vi "final_lucas_valeria.vi"() -> ()   [LabVIEW 2017]
uses:
  <vilib>/ErrorRing/Error Ring.xnode
  final.ctl
  <vilib>/Utility/file.llb/Read Delimited Spreadsheet (string).vi
panel:
  out "Decodificar":string
  out "substring":string
  out "cabecera":bool
  out "x = y?":bool
  out "led3":bool
  out "led2":bool
  out "led1":bool
  in  "Umbral min3":dbl
  in  "Umbral max3":dbl
  in  "Umbral min2":dbl
  in  "Umbral max2":dbl
  in  "Umbral min1":dbl
  in  "Umbral max1":dbl
  out "pt100":dbl(knob) scale=0.0..100.0
  out "ntc":dbl(knob) scale=0.0..100.0
  out "lm35":dbl(knob) scale=0.0..150.0
  out "Waveform Chart":cluster{"lm35":dbl, "ntc":dbl}(graph)
  out "NTC":dbl=25.0 format="%0.2f"
  out "lM35":dbl
  out "Dato3":dbl
  out "Dato2":dbl
  out "verifica_cheacksum":string
  out "Dato_Act":string
  out "size":i32
  out "CHECKSUM":string
  out "Desconexión":bool
  out "Hora de desconexión":string
  out "Stop":bool
  in  "BaudRate":i32(ring) items=["9600"=9600, "11520"=11520]
  out "error out":errorcluster
  out "On":bool
  out "Recibiendo datos":bool
  out "Datos Sensores":string
  in  "Close":bool
  in  "Open":bool
  in  "Port":string(combo)
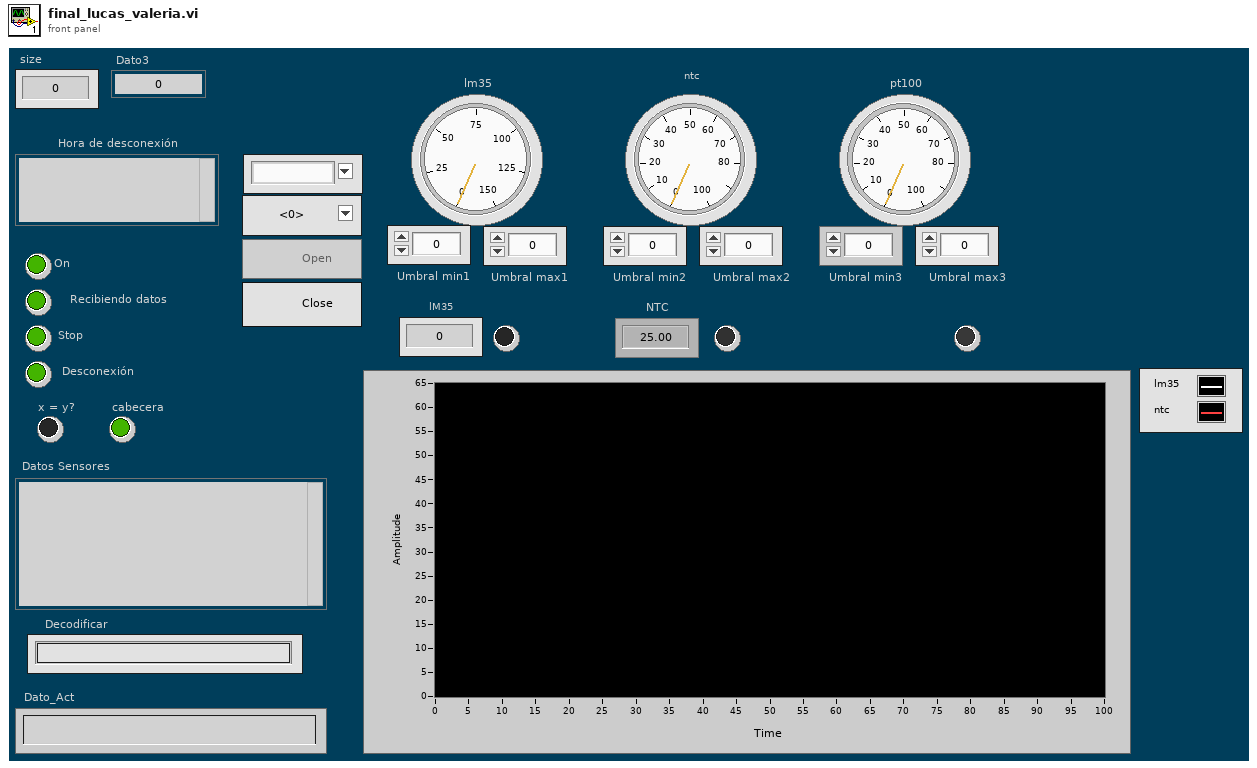
[diagram p1: front panel]
types:
  T1 = typedef "final.ctl" = enum16{"verificar", "verificar2", "sacar_datos", "alarma1", "alarma2", "alarma3"}
  T2 = enum8{"Enabled", "Disabled", "Disabled and Grayed Out"}
  T3 = enum16{"open", "replace", "create", "open or create", "replace or create", "replace or create with confirmation"}
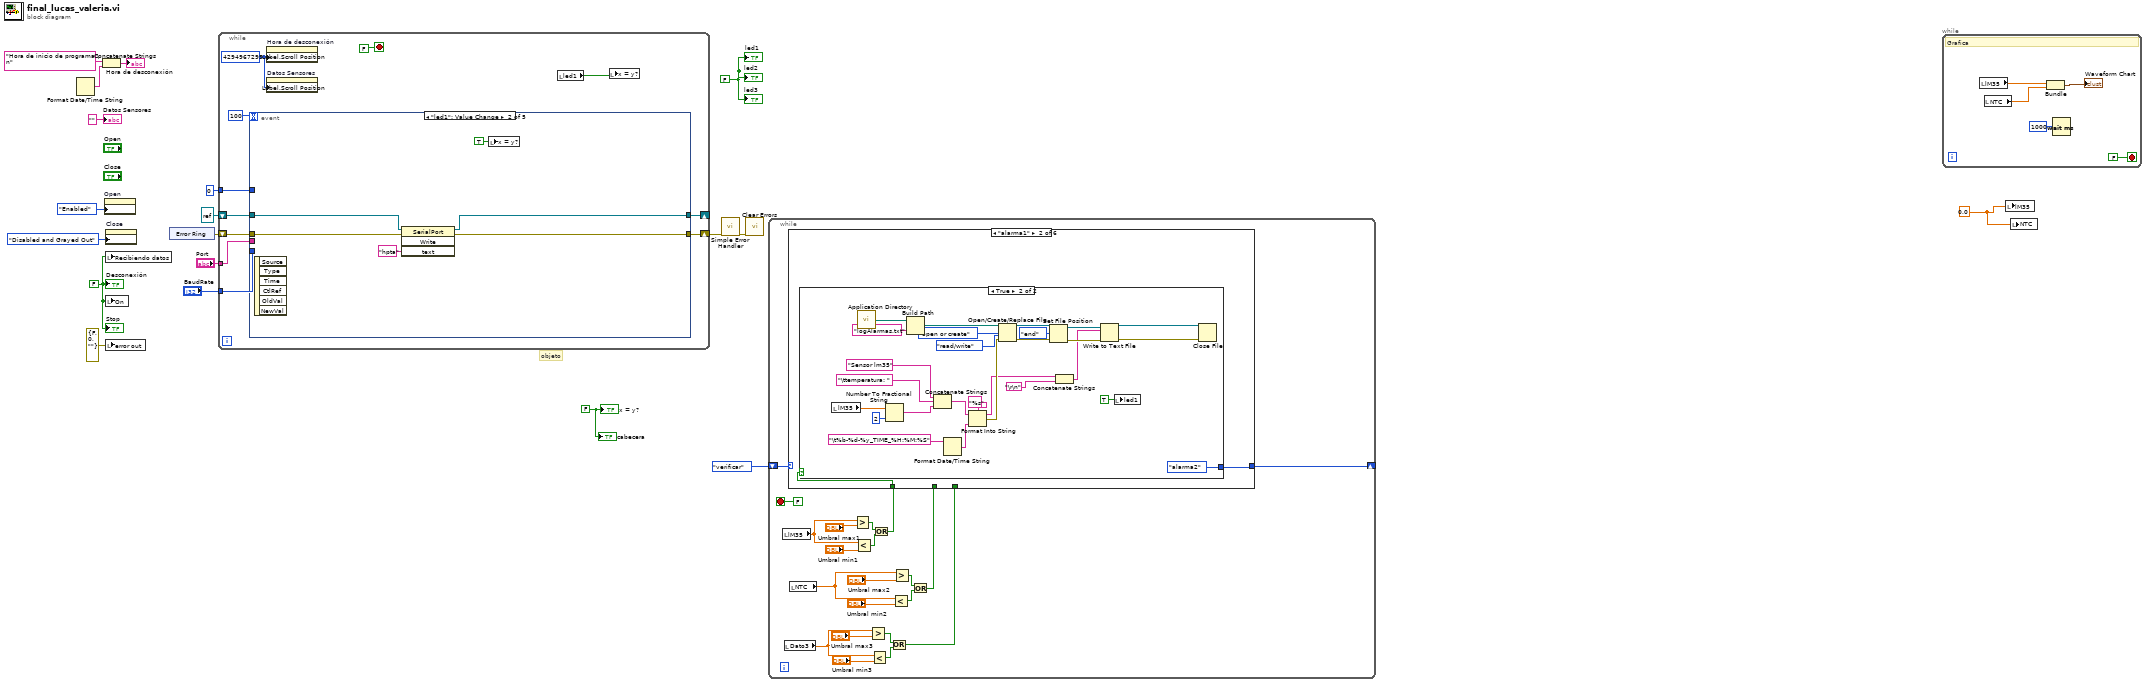
[diagram p0: block diagram]
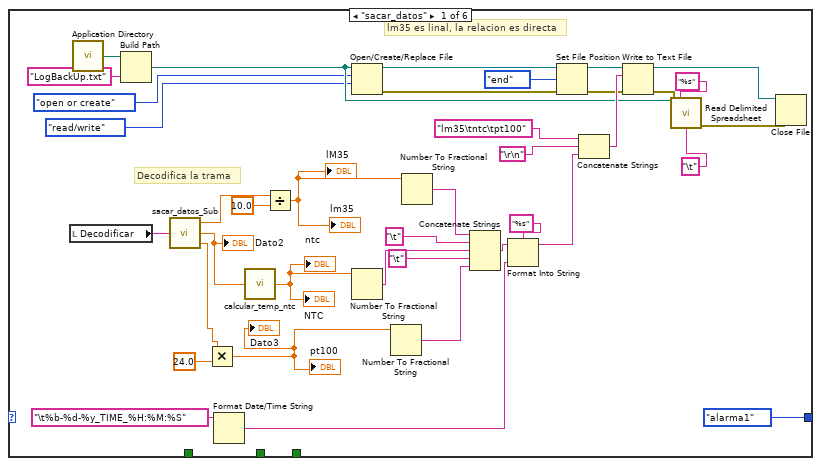
[diagram p2: hidden frame]
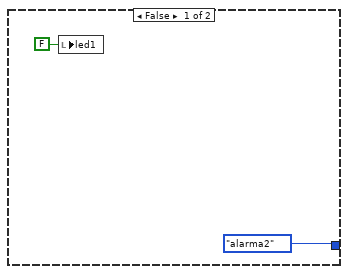
[diagram p3: hidden frame]
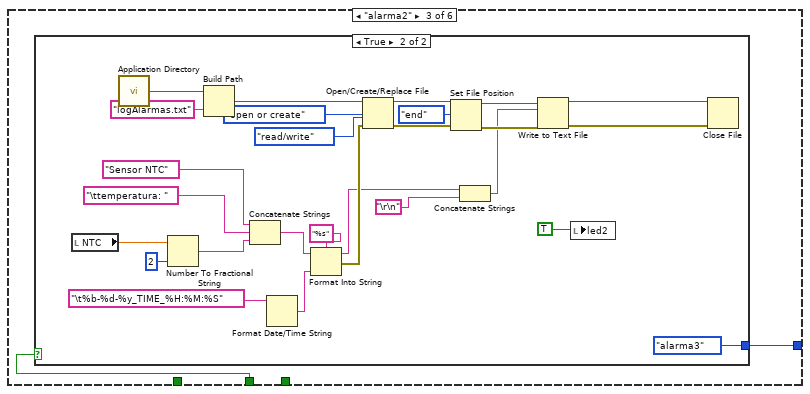
[diagram p4: hidden frame]
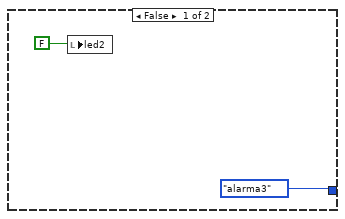
[diagram p5: hidden frame]
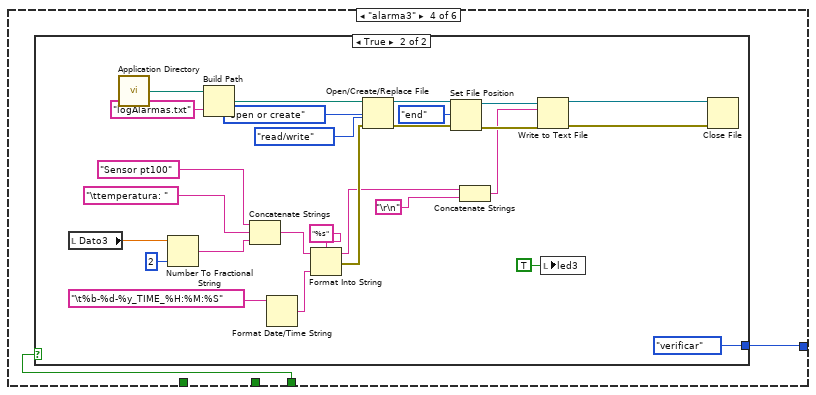
[diagram p6: hidden frame]
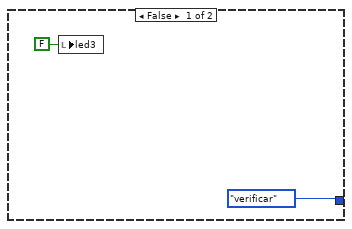
[diagram p7: hidden frame]
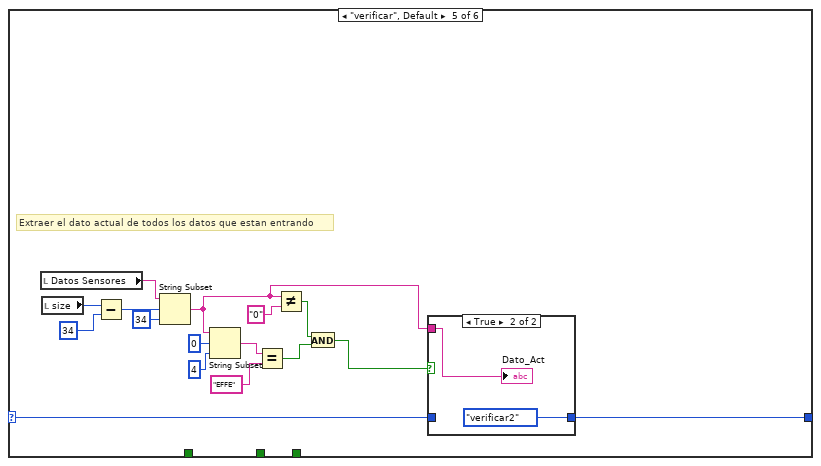
[diagram p8: hidden frame]
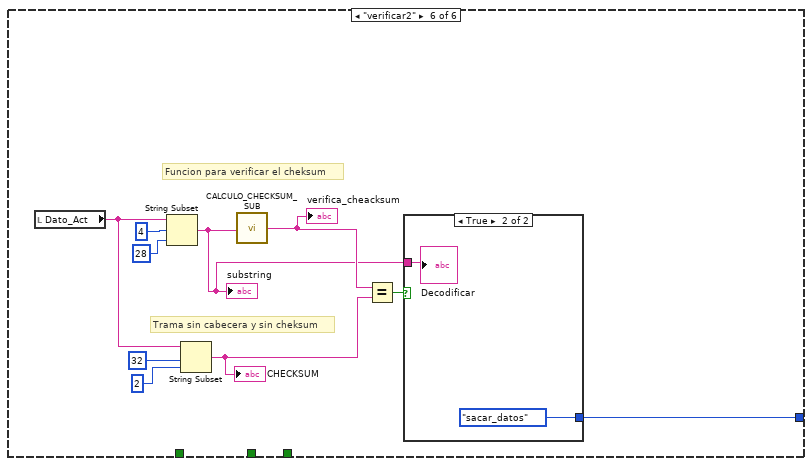
[diagram p10: hidden frame]
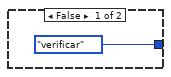
[diagram p11: hidden frame]
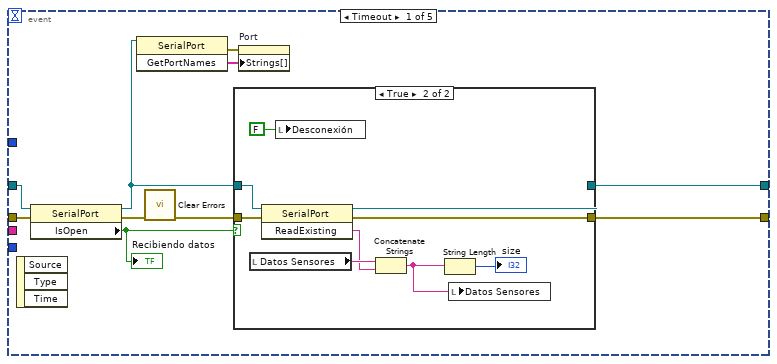
[diagram p12: hidden frame]
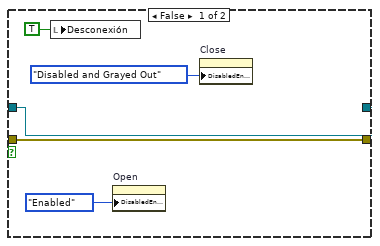
[diagram p13: hidden frame]
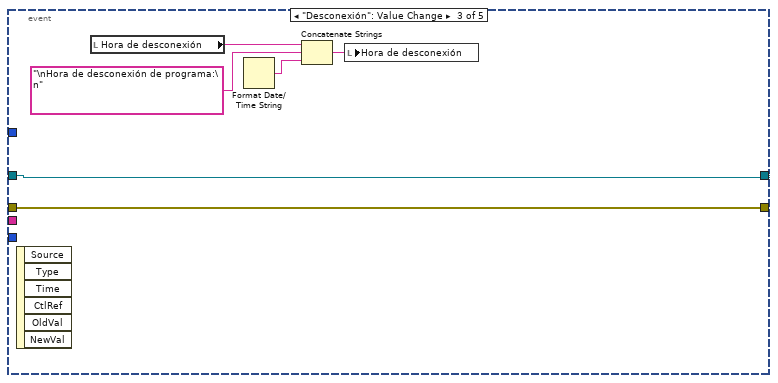
[diagram p14: hidden frame]
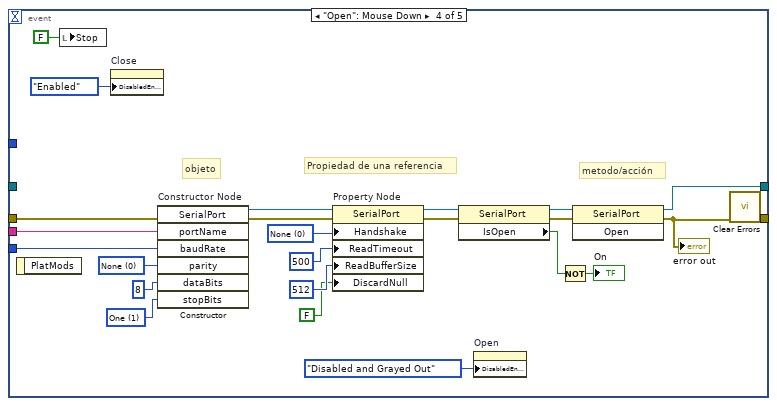
[diagram p15: hidden frame]
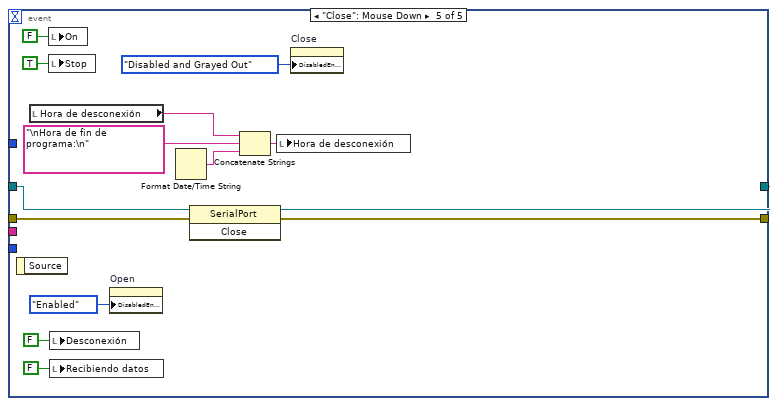
[diagram p16: hidden frame]
diagram:
  w1 = FALSE ("x = y?")
  w3 = FALSE ("led1")
  w4 = sgl 0.0 ("lm35")
  w2 = FALSE ("Recibiendo datos")
  # "objeto"
  n1 = Format Date/Time String() -> (date/time string=w9:string)  [unwired: 3 in]
  n2 = Concatenate Strings("Hora de inicio de programa:\n" ("String"), w9) -> (→"Hora de desconexión":string)
  n3 = property on="Open" class="Bool (strict)"("DisabledEnum"=T2."Enabled" ("Disabled")) -> ()  [unwired: 2 in, 2 out]
  n4 = property on="Close" class="Bool (strict)"("DisabledEnum"=T2."Disabled and Grayed Out" ("Disabled")) -> ()  [unwired: 2 in, 2 out]
  n5 = local write "Recibiendo datos"(w2) -> ()
  n6 = local write "On"(w2) -> ()
  n7 = local write "error out"(errorcluster {"status"=FALSE, "code"=0, "source"=""} ("error out")) -> ()
  n8 = xnode "Error Ring"() -> ("error out"=w7:errorcluster)
  n9 = while {
    tunnel: "Port" -> [w29]
    shift-right: [w27] -> _
    shift-left: refnum<k24> refnum ("reference") -> [w28]
    shift-right: [w26] -> w18
    shift-left: w7 -> [w21]
    tunnel: "BaudRate" -> [w24]
    tunnel: 0 -> [w22]
    stop <- FALSE stop-if-true
    w23 = u32 4294967295 ("Label.Scroll Position")
    n10 = event shown="[1] \"led1\": Value Change" {
      selector: _ -> [_ _ _ _ _]
      dyn-events: _ -> [_ _ _ _ _]
      timeout: 100 -> [_ _ _ _ _]
      tunnel: w29 -> [_ _ _ w90 _]
      tunnel: [w34 w55 w61 w89 w99] -> w26
      tunnel: [w35 w56 w62 w88 w100] -> w27
      tunnel: w28 -> [w32 w57 w62 _ w102]
      tunnel: w21 -> [w33 w58 w61 w87 w101]
      tunnel: w24 -> [_ _ _ w73 _]
      tunnel: w22 -> [_ _ _ _ _]
      event Timeout {
        n11 = event-data() -> ()  [unwired: 1 in, 3 out]
        n12 = property class="SerialPort"(reference=w32, error in=w33) -> (reference out=w37:refnum<k24>, error out=w36:errorcluster, "IsOpen"=w31:bool)
        "Recibiendo datos" <- w31
        n13 = invoke class="SerialPort" method="GetPortNames"(reference=w37) -> (error out=w40:errorcluster, "GetPortNames"=w39:string[])  [unwired: 2 in, 1 out]
        n14 = call <vilib>:"Clear Errors.vi"("error in (no error)"=w36) -> ("error out"=w38:errorcluster)  [unwired: 5 in, 1 out]
        n15 = case shown="True" w31 {
          tunnel: w37 -> [w45 w49]
          tunnel: w38 -> [w44 w54]
          tunnel: [w45 w51] -> w35
          tunnel: [w44 w50] -> w34
          frame False {
            n16 = local write "Desconexión"(TRUE ("Error de desconexión")) -> ()
            n17 = property on="Open" class="Bool (strict)"("DisabledEnum"=T2."Enabled" ("Disabled")) -> ()  [unwired: 2 in, 2 out]
            n18 = property on="Close" class="Bool (strict)"("DisabledEnum"=T2."Disabled and Grayed Out" ("Disabled")) -> ()  [unwired: 2 in, 2 out]
          }
          frame True {
            n19 = local read "Datos Sensores"() -> (w53:string)
            n20 = invoke class="SerialPort" method="ReadExisting"(reference=w49, error in=w54) -> (reference out=w51:refnum<k24>, error out=w50:errorcluster, "ReadExisting"=w52:string)  [unwired: 1 in]
            n21 = local write "Desconexión"(FALSE ("Error de desconexión")) -> ()
            n22 = Concatenate Strings(w53, w52) -> (w46:string)
            n23 = String Length(string=w46) -> (length=→"size":i32)
            n24 = local write "Datos Sensores"(w46) -> ()
          }
        }
        n25 = property on="Port" class="CmbBox"(error in=w40, "Strings[]"=w39) -> ()  [unwired: 1 in, 2 out]
      }
      event "led1": Value Change {
        n26 = event-data() -> ()  [unwired: 1 in, 6 out]
        n27 = invoke class="SerialPort" method="Write"(reference=w57, error in=w58, "text"="hpta") -> (reference out=w56:refnum<k24>, error out=w55:errorcluster)  [unwired: 1 in, 2 out]
        n28 = local write "x = y?"(TRUE ("x = y?")) -> ()
      }
      event "Desconexión": Value Change {
        n29 = event-data() -> ()  [unwired: 1 in, 6 out]
        n30 = local read "Hora de desconexión"() -> (w64:string)
        n31 = Format Date/Time String() -> (date/time string=w65:string)  [unwired: 3 in]
        n32 = Concatenate Strings(w64, "\nHora de desconexión de programa:\n" ("String"), w65) -> (w66:string)
        n33 = local write "Hora de desconexión"(w66) -> ()
      }
      event "Open": Mouse Down {
        w67 = 1 items=["None", "One", "Two", "OnePointFive"] ("stopBits")
        w69 = 0 items=["None", "Odd", "Even", "Mark", "Space"] ("parity")
        w84 = 0 items=["None", "XOnXOff", "RequestToSend", "RequestToSendXOnXOff"] ("Handshake")
        # "Propiedad de una referencia"
        # "metodo/acción"
        # "objeto"
        n34 = event-data() -> ()  [unwired: 1 in, 1 out]
        n35 = local write "Stop"(FALSE ("Boolean")) -> ()
        n36 = property on="Close" class="Bool (strict)"("DisabledEnum"=T2."Enabled" ("Disabled")) -> ()  [unwired: 2 in, 2 out]
        n37 = constructor on="Constructor Node" class="SerialPort"(error in=w87, "portName"=w90, "baudRate"=w73, "parity"=w69, "dataBits"=8, "stopBits"=w67) -> (reference out=w85:refnum<k24>, error out=w80:errorcluster)  [unwired: 2 in, 6 out]
        n38 = property on="Property Node" class="SerialPort"(reference=w85, error in=w80, "Handshake"=w84, "ReadTimeout"=500, "ReadBufferSize"=512, "DiscardNull"=FALSE) -> (reference out=w78:refnum<k24>, error out=w77:errorcluster)
        n39 = property class="SerialPort"(reference=w78, error in=w77) -> (reference out=w76:refnum<k24>, error out=w75:errorcluster, "IsOpen"=w72:bool)
        n40 = property on="Open" class="Bool (strict)"("DisabledEnum"=T2."Disabled and Grayed Out" ("Disabled")) -> ()  [unwired: 2 in, 2 out]
        n41 = Not(x=w72) -> (.not. x?=→"On":bool)
        n42 = invoke class="SerialPort" method="Open"(reference=w76, error in=w75) -> (reference out=w88:refnum<k24>, error out=w74:errorcluster)  [unwired: 1 in, 1 out]
        "error out" <- w74
        n43 = call <vilib>:"Clear Errors.vi"("error in (no error)"=w74) -> ("error out"=w89:errorcluster)  [unwired: 5 in, 1 out]
      }
      event "Close": Mouse Down {
        n44 = event-data() -> ()  [unwired: 1 in, 1 out]
        n45 = local read "Hora de desconexión"() -> (w91:string)
        n46 = local write "On"(FALSE ("Boolean")) -> ()
        n47 = local write "Stop"(TRUE ("Boolean")) -> ()
        n48 = local write "Desconexión"(FALSE ("Boolean")) -> ()
        n49 = local write "Recibiendo datos"(FALSE ("Boolean")) -> ()
        n50 = property on="Open" class="Bool (strict)"("DisabledEnum"=T2."Enabled" ("Disabled")) -> ()  [unwired: 2 in, 2 out]
        n51 = Format Date/Time String() -> (date/time string=w93:string)  [unwired: 3 in]
        n52 = invoke class="SerialPort" method="Close"(reference=w102, error in=w101) -> (reference out=w100:refnum<k24>, error out=w99:errorcluster)  [unwired: 1 in, 1 out]
        n53 = Concatenate Strings(w91, "\nHora de fin de programa:\n" ("String"), w93) -> (w94:string)
        n54 = local write "Hora de desconexión"(w94) -> ()
        n55 = property on="Close" class="Bool (strict)"("DisabledEnum"=T2."Disabled and Grayed Out" ("Disabled")) -> ()  [unwired: 2 in, 2 out]
      }
    }
    n56 = property on="Hora de desconexión" class="Str"("Label.Scroll Position"=w23) -> ()  [unwired: 2 in, 2 out]
    n57 = property on="Datos Sensores" class="Str"("Label.Scroll Position"=w23) -> ()  [unwired: 2 in, 2 out]
    n58 = local read "led1"() -> (w20:bool)
    n59 = local write "x = y?"(w20) -> ()
  }
  n60 = call <vilib>:"Simple Error Handler.vi"("error in (no error)"=w18) -> ("error out"=w17:errorcluster)  [unwired: 4 in, 4 out]
  n61 = call <vilib>:"Clear Errors.vi"("error in (no error)"=w17) -> ()  [unwired: 5 in, 2 out]
  n62 = while {
    shift-right: [w123] -> _
    shift-left: final."verificar" -> [w124]
    stop <- FALSE stop-if-true
    n63 = local read "lM35"() -> (w118:dbl)
    n64 = local read "Dato3"() -> (w109:dbl)
    n65 = local read "NTC"() -> (w116:dbl)
    n66 = Greater?(x=w118, y="Umbral max1") -> (0:w119:bool)
    n67 = Less?(x=w118, y="Umbral min1") -> (x < y?=w120:bool)
    n68 = Greater?(x=w109, y="Umbral max3") -> (0:w107:bool)
    n69 = Less?(x=w109, y="Umbral min3") -> (x < y?=w106:bool)
    n70 = Or(x=w119, y=w120) -> (x .or. y?=w117:bool)
    n71 = Or(x=w107, y=w106) -> (x .or. y?=w105:bool)
    n72 = Less?(x=w116, y="Umbral min2") -> (x < y?=w112:bool)
    n73 = Greater?(x=w116, y="Umbral max2") -> (0:w113:bool)
    n74 = Or(x=w113, y=w112) -> (x .or. y?=w111:bool)
    n75 = case shown="\"alarma1\"" w124 {
      selector: w124 -> [_ _ _ _ w270 _]
      tunnel: [final."alarma1" w164 w195 w227 w269 w280] -> w123
      tunnel: w117 -> [_ w165 _ _ _ _]
      tunnel: w111 -> [_ _ w196 _ _ _]
      tunnel: w105 -> [_ _ _ w226 _ _]
      frame "sacar_datos" {
        # "Decodifica la trama"
        # "lm35 es linal, la relacion es directa"
        n76 = local read "Decodificar"() -> (w126:string)
        n77 = call <vilib>:"Application Directory.vi"() -> ("Application Directory"=w158:path)
        n78 = Build Path(base path=w158, name or relative path="LogBackUp.txt") -> (appended path=w147:path)
        n79 = call "sacar_datos_Sub.vi"("Dato"=w126) -> ("Dato3"=w129:dbl, "Dato2"=w163:dbl, "Dato1"=w161:dbl)  [unwired: 2 in]
        "Dato2" <- w163
        n80 = Multiply(x=w129, y=24.0) -> (x*y=w127:dbl)
        "Dato3" <- w127
        "pt100" <- w127
        n81 = Format Date/Time String(time format string (%c)="\t%b-%d-%y_TIME_%H:%M:%S") -> (date/time string=w143:string)  [unwired: 2 in]
        n82 = call "calcular_temp_ntc.vi"("Vin"=w163) -> ("temp_ntc"=w141:dbl)
        "NTC" <- w141
        "ntc" <- w141
        n83 = Divide(x=w161, y=10.0) -> (x/y=w142:dbl)
        "lM35" <- w142
        "lm35" <- w142
        n84 = Open/Create/Replace File(file path (use dialog)=w147, operation (0:open)=T3."open or create", access (0:read/write)=enum16{"read/write", "read-only", "write-only"}."read/write") -> (refnum out=w149:refnum<file>, error out=w150:errorcluster)  [unwired: 3 in, 1 out]
        n85 = Number To Fractional String(number=w141) -> (F-format string=w138:string)  [unwired: 3 in]
        n86 = Number To Fractional String(number=w127) -> (F-format string=w136:string)  [unwired: 3 in]
        n87 = Number To Fractional String(number=w142) -> (F-format string=w140:string)  [unwired: 3 in]
        n88 = Concatenate Strings(w140, "\t" ("format string"), w138, "\t" ("format string"), w136) -> (w135:string)
        n89 = Format Into String(format string="%s", initial string=w135, w143) -> (resulting string=w132:string)  [unwired: 1 in, 1 out]
        n90 = Set File Position(refnum=w149, from (0:start)=enum16{"start", "end", "current"}."end", error in=w150) -> (refnum out=w148:refnum<file>, error out=w151:errorcluster)  [unwired: 1 in]
        n91 = Concatenate Strings("lm35\tntc\tpt100" ("format string"), "\r\n", w132) -> (w157:string)
        n92 = Write to Text File(file (use dialog)=w148, text=w157, error in=w151) -> (refnum out=w156:refnum<file>, error out=w154:errorcluster)  [unwired: 1 in, 1 out]
        n93 = call-poly <vilib>:"Read Delimited Spreadsheet.vi"("file path (dialog if empty)"=w147, "format (%s)"="%s", "error in (no error)"=w154, "delimiter (\\t)"="\t" ("delimiter (\\t)")) -> ("error out"=w155:errorcluster)  [unwired: 6 in, 5 out]
        n94 = Close File(refnum=w156, error in=w155) -> ()  [unwired: 2 out]
      }
      frame "alarma1" {
        n95 = case shown="True" w165 {
          tunnel: [final."alarma2" final."alarma2"] -> w164
          frame False {
            n96 = local write "led1"(FALSE ("led1")) -> ()
          }
          frame True {
            n97 = local read "lM35"() -> (w170:dbl)
            n98 = call <vilib>:"Application Directory.vi"() -> ("Application Directory"=w194:path)
            n99 = Number To Fractional String(number=w170, precision (6)=i16 2) -> (F-format string=w173:string)  [unwired: 2 in]
            n100 = Build Path(base path=w194, name or relative path="logAlarmas.txt") -> (appended path=w193:path)
            n101 = Concatenate Strings("Sensor lm35" ("format string"), "\ttemperatura: " ("format string"), w173) -> (w172:string)
            n102 = Format Date/Time String(time format string (%c)="\t%b-%d-%y_TIME_%H:%M:%S") -> (date/time string=w179:string)  [unwired: 2 in]
            n103 = Format Into String(format string="%s", initial string=w172, w179) -> (resulting string=w177:string, error out=w181:errorcluster)  [unwired: 1 in]
            n104 = Open/Create/Replace File(file path (use dialog)=w193, error in=w181, operation (0:open)=T3."open or create", access (0:read/write)=enum16{"read/write", "read-only", "write-only"}."read/write") -> (refnum out=w189:refnum<file>, error out=w188:errorcluster)  [unwired: 2 in, 1 out]
            n105 = Set File Position(refnum=w189, from (0:start)=enum16{"start", "end", "current"}."end", error in=w188) -> (refnum out=w186:refnum<file>, error out=w185:errorcluster)  [unwired: 1 in]
            n106 = Concatenate Strings(w177, "\r\n") -> (w176:string)
            n107 = Write to Text File(file (use dialog)=w186, text=w176, error in=w185) -> (refnum out=w184:refnum<file>, error out=w183:errorcluster)  [unwired: 1 in, 1 out]
            n108 = local write "led1"(TRUE ("led1")) -> ()
            n109 = Close File(refnum=w184, error in=w183) -> ()  [unwired: 2 out]
          }
        }
      }
      frame "alarma2" {
        n110 = case shown="True" w196 {
          tunnel: [final."alarma3" final."alarma3"] -> w195
          frame False {
            n111 = local write "led2"(FALSE ("led1")) -> ()
          }
          frame True {
            n112 = local read "NTC"() -> (w199:dbl)
            n113 = call <vilib>:"Application Directory.vi"() -> ("Application Directory"=w225:path)
            n114 = Number To Fractional String(number=w199, precision (6)=i16 2) -> (F-format string=w204:string)  [unwired: 2 in]
            n115 = Build Path(base path=w225, name or relative path="logAlarmas.txt") -> (appended path=w224:path)
            n116 = Concatenate Strings("Sensor NTC" ("format string"), "\ttemperatura: " ("format string"), w204) -> (w203:string)
            n117 = Format Date/Time String(time format string (%c)="\t%b-%d-%y_TIME_%H:%M:%S") -> (date/time string=w210:string)  [unwired: 2 in]
            n118 = Format Into String(format string="%s", initial string=w203, w210) -> (resulting string=w208:string, error out=w212:errorcluster)  [unwired: 1 in]
            n119 = Open/Create/Replace File(file path (use dialog)=w224, error in=w212, operation (0:open)=T3."open or create", access (0:read/write)=enum16{"read/write", "read-only", "write-only"}."read/write") -> (refnum out=w220:refnum<file>, error out=w219:errorcluster)  [unwired: 2 in, 1 out]
            n120 = Set File Position(refnum=w220, from (0:start)=enum16{"start", "end", "current"}."end", error in=w219) -> (refnum out=w217:refnum<file>, error out=w216:errorcluster)  [unwired: 1 in]
            n121 = Concatenate Strings(w208, "\r\n") -> (w207:string)
            n122 = Write to Text File(file (use dialog)=w217, text=w207, error in=w216) -> (refnum out=w215:refnum<file>, error out=w214:errorcluster)  [unwired: 1 in, 1 out]
            n123 = local write "led2"(TRUE ("led1")) -> ()
            n124 = Close File(refnum=w215, error in=w214) -> ()  [unwired: 2 out]
          }
        }
      }
      frame "alarma3" {
        n125 = case shown="True" w226 {
          tunnel: [final."verificar" final."verificar"] -> w227
          frame False {
            n126 = local write "led3"(FALSE ("led3")) -> ()
          }
          frame True {
            n127 = local read "Dato3"() -> (w231:dbl)
            n128 = call <vilib>:"Application Directory.vi"() -> ("Application Directory"=w256:path)
            n129 = Number To Fractional String(number=w231, precision (6)=i16 2) -> (F-format string=w235:string)  [unwired: 2 in]
            n130 = Build Path(base path=w256, name or relative path="logAlarmas.txt") -> (appended path=w255:path)
            n131 = Concatenate Strings("Sensor pt100" ("format string"), "\ttemperatura: " ("format string"), w235) -> (w234:string)
            n132 = Format Date/Time String(time format string (%c)="\t%b-%d-%y_TIME_%H:%M:%S") -> (date/time string=w241:string)  [unwired: 2 in]
            n133 = Format Into String(format string="%s", initial string=w234, w241) -> (resulting string=w239:string, error out=w243:errorcluster)  [unwired: 1 in]
            n134 = Open/Create/Replace File(file path (use dialog)=w255, error in=w243, operation (0:open)=T3."open or create", access (0:read/write)=enum16{"read/write", "read-only", "write-only"}."read/write") -> (refnum out=w251:refnum<file>, error out=w250:errorcluster)  [unwired: 2 in, 1 out]
            n135 = Set File Position(refnum=w251, from (0:start)=enum16{"start", "end", "current"}."end", error in=w250) -> (refnum out=w248:refnum<file>, error out=w247:errorcluster)  [unwired: 1 in]
            n136 = Concatenate Strings(w239, "\r\n") -> (w238:string)
            n137 = Write to Text File(file (use dialog)=w248, text=w238, error in=w247) -> (refnum out=w246:refnum<file>, error out=w245:errorcluster)  [unwired: 1 in, 1 out]
            n138 = local write "led3"(TRUE ("led3")) -> ()
            n139 = Close File(refnum=w246, error in=w245) -> ()  [unwired: 2 out]
          }
        }
      }
      frame "verificar", Default {
        # "Extraer el dato actual de todos los datos que estan entrando"
        n140 = local read "Datos Sensores"() -> (w260:string)
        n141 = local read "size"() -> (w272:i32)
        n142 = Subtract(x=w272, y=34) -> (x-y=w262:i32)
        n143 = String Subset(string=w260, offset (0)=w262, length (rest)=34 ("length (rest)")) -> (substring=w257:string)
        n144 = String Subset(string=w257, offset (0)=0, length (rest)=4 ("length (rest)")) -> (substring=w264:string)
        n145 = Equal?(x=w264, y="EFFE") -> (x = y?=w259:bool)
        n146 = Not Equal?(x=w257, y="0") -> (x != y?=w258:bool)
        n147 = And(x=w258, y=w259) -> (x .and. y?=w268:bool)
        n148 = case shown="True" w268 {
          tunnel: w270 -> [w273 _]
          tunnel: [w273 final."verificar2"] -> w269
          tunnel: w257 -> [_ w274]
          frame False {
          }
          frame True {
            "Dato_Act" <- w274
          }
        }
      }
      frame "verificar2" {
        # "Trama sin cabecera y sin cheksum"
        # "Funcion para verificar el cheksum"
        n149 = local read "Dato_Act"() -> (w279:string)
        n150 = String Subset(string=w279, offset (0)=4, length (rest)=28 ("length (rest)")) -> (substring=w276:string)
        "substring" <- w276
        n151 = String Subset(string=w279, offset (0)=32, length (rest)=2 ("length (rest)")) -> (substring=w278:string)
        "CHECKSUM" <- w278
        n152 = call "CALCULO_CHECKSUM_SUB.vi"("DATOS"=w276) -> ("verificado"=w277:string)
        "verifica_cheacksum" <- w277
        n153 = Equal?(x=w277, y=w278) -> (x = y?=w281:bool)
        n154 = case shown="True" w281 {
          tunnel: [final."verificar" final."sacar_datos"] -> w280
          tunnel: w276 -> [_ w287]
          frame False {
          }
          frame True {
            "Decodificar" <- w287
          }
        }
      }
    }
  }
  n155 = while {
    stop <- FALSE stop-if-true
    # "Grafica"
    n156 = local read "lM35"() -> (w292:dbl)
    n157 = local read "NTC"() -> (w291:dbl)
    n158 = Bundle("lM35"=w292, "NTC"=w291) -> (→"Waveform Chart":cluster{"lM35":dbl, "NTC":dbl})  [unwired: 1 in]
    n159 = Wait (ms)(milliseconds to wait=u32 1000) -> ()  [unwired: 1 out]
  }
  n160 = local write "lM35"(w4) -> ()
  n161 = local write "NTC"(w4) -> ()
  "Datos Sensores" <- "" ("String")
  "Stop" <- w2
  "Desconexión" <- w2
  "led1" <- w3
  "led2" <- w3
  "led3" <- w3
  "x = y?" <- w1
  "cabecera" <- w1
